vi "ConfigParseMultipleMicroscopes.vi"(8 "error in (no error)":errorcluster, 10 "node result array":refnum<k20>[](array[refnum])) -> (0 "error out":errorcluster, 3 "Array":string[][](array[string]))   [LabVIEW 2018, in "Config.lvlib"]
uses:
  Config.lvlib
  <vilib>/xml/Close Reference(Node).vi
  <vilib>/xml/NI_XML.lvlib
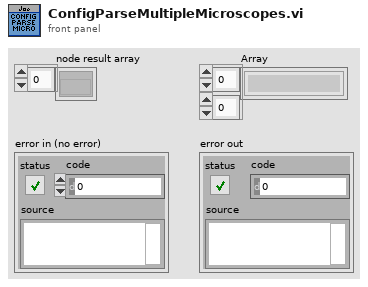
[diagram p1: front panel]
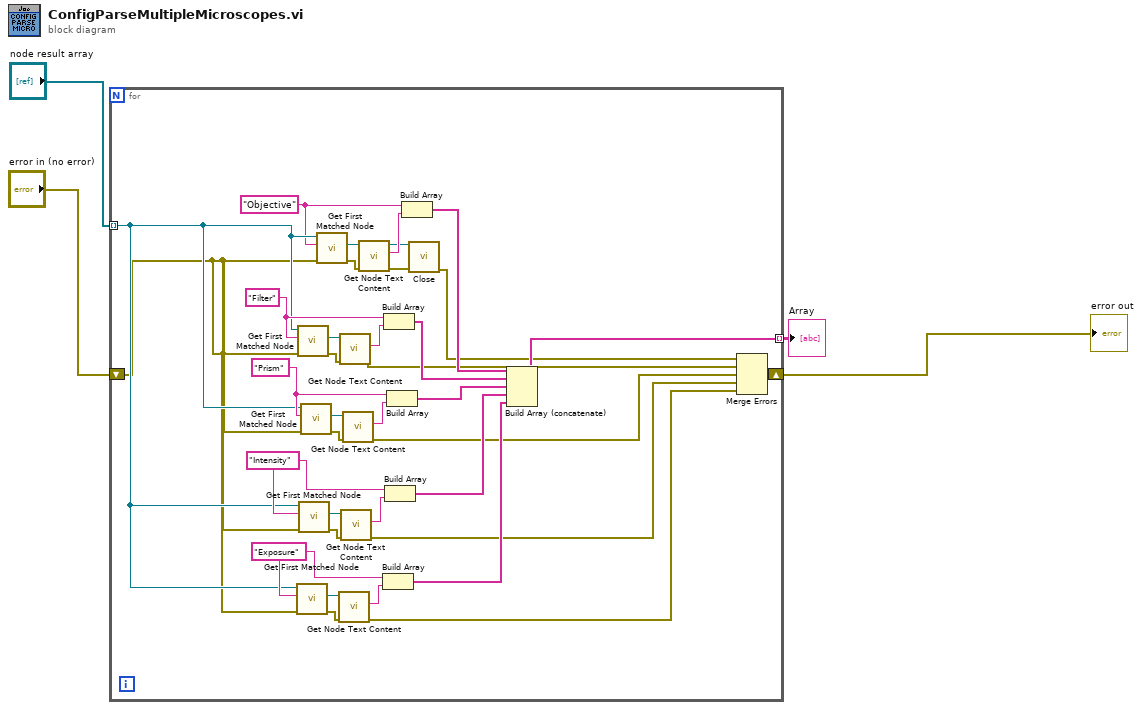
[diagram p0: block diagram]
diagram:
  n1 = for {
    tunnel: "node result array" -> [w12] mode=indexing
    tunnel: [w10] -> w3 mode=indexing
    shift-right: [w9] -> w4
    shift-left: "error in (no error)" -> [w11]
    w25 = "Exposure" ("XPath expression")
    w30 = "Intensity" ("XPath expression")
    w33 = "Prism" ("XPath expression")
    w36 = "Filter" ("XPath expression")
    w5 = "Objective" ("XPath expression")
    n2 = call <vilib>:"Get First Matched Node.vi"("error in (no error)"=w11, "XPath expression"=w25, "node in"=w12) -> ("error out"=w17:errorcluster, "node result"=w26:refnum<k20>)  [unwired: 6 in, 1 out]
    n3 = call <vilib>:"Get First Matched Node.vi"("error in (no error)"=w11, "XPath expression"=w36, "node in"=w12) -> ("error out"=w20:errorcluster, "node result"=w37:refnum<k20>)  [unwired: 6 in, 1 out]
    n4 = call <vilib>:"Get First Matched Node.vi"("error in (no error)"=w11, "XPath expression"=w30, "node in"=w12) -> ("error out"=w18:errorcluster, "node result"=w31:refnum<k20>)  [unwired: 6 in, 1 out]
    n5 = call <vilib>:"Get First Matched Node.vi"("error in (no error)"=w11, "XPath expression"=w33, "node in"=w12) -> ("error out"=w19:errorcluster, "node result"=w34:refnum<k20>)  [unwired: 6 in, 1 out]
    n6 = call <vilib>:"Get First Matched Node.vi"("error in (no error)"=w11, "XPath expression"=w5, "node in"=w12) -> ("error out"=w21:errorcluster, "node result"=w40:refnum<k20>)  [unwired: 6 in, 1 out]
    n7 = call <vilib>:"Get Node Text Content.vi"("error in (no error)"=w17, "node in"=w26) -> ("error out"=w13:errorcluster, "node text"=w24:string)  [unwired: 7 in, 1 out]
    n8 = call <vilib>:"Get Node Text Content.vi"("error in (no error)"=w20, "node in"=w37) -> ("error out"=w16:errorcluster, "node text"=w35:string)  [unwired: 7 in, 1 out]
    n9 = call <vilib>:"Get Node Text Content.vi"("error in (no error)"=w18, "node in"=w31) -> ("error out"=w14:errorcluster, "node text"=w29:string)  [unwired: 7 in, 1 out]
    n10 = call <vilib>:"Get Node Text Content.vi"("error in (no error)"=w19, "node in"=w34) -> ("error out"=w15:errorcluster, "node text"=w32:string)  [unwired: 7 in, 1 out]
    n11 = call <vilib>:"Get Node Text Content.vi"("error in (no error)"=w21, "node in"=w40) -> ("error out"=w7:errorcluster, "node text"=w39:string, "node out"=w8:refnum<k20>)  [unwired: 7 in]
    n12 = Build Array(w25, w24) -> (w22:string[])
    n13 = Build Array(w36, w35) -> (w28:string[])
    n14 = Build Array(w30, w29) -> (w23:string[])
    n15 = Build Array(w33, w32) -> (w27:string[])
    n16 = Build Array(w5, w39) -> (w38:string[])
    n17 = call-poly <vilib>:"Close.vi"("error in (no error)"=w7, "node"=w8) -> ("error out"=w6:errorcluster)  [unwired: 7 in]
    n18 = Build Array (concatenate)(w38, w28, w27, w23, w22) -> (w10:string[])
    n19 = Merge Errors(w6, w16, w15, w14, w13) -> (w9:errorcluster)
  }
  "error out" <- w4
  "Array" <- w3
